vi "bapsf_motion_lv.vi"(4 "error in":errorcluster, 6 "Request data":variant, 7 "Request":string) -> (0 "error out":errorcluster, 2 "Response data":variant)   [LabVIEW 2018]
panel:
  out "Python session":refnum<k35>
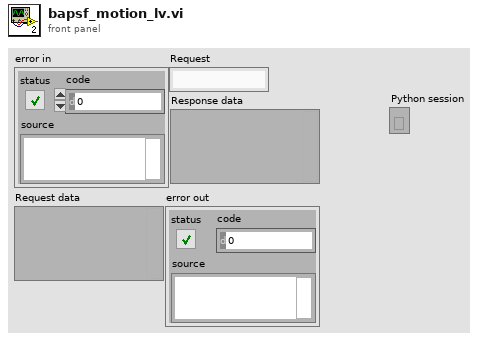
[diagram p1: front panel]
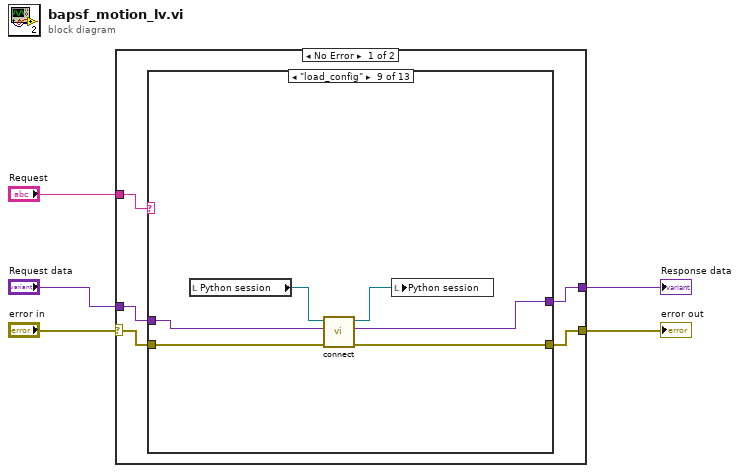
[diagram p0: block diagram]
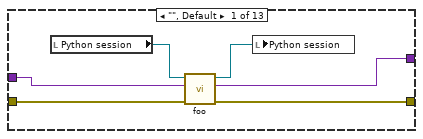
[diagram p2: hidden frame]
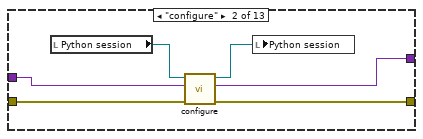
[diagram p3: hidden frame]
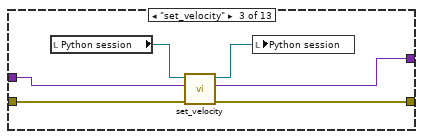
[diagram p4: hidden frame]
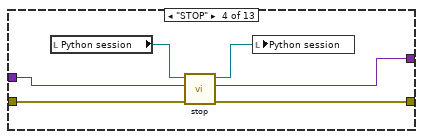
[diagram p5: hidden frame]
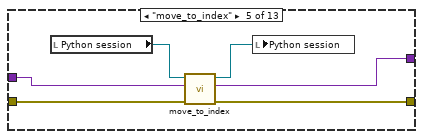
[diagram p6: hidden frame]
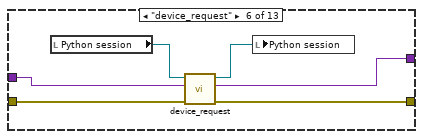
[diagram p7: hidden frame]
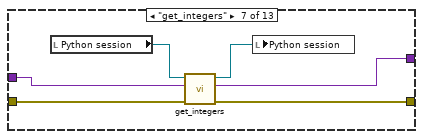
[diagram p8: hidden frame]
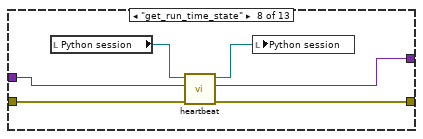
[diagram p9: hidden frame]
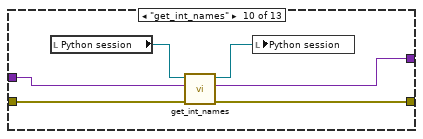
[diagram p10: hidden frame]
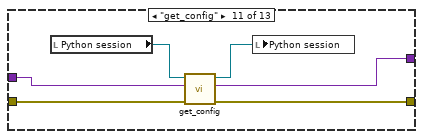
[diagram p11: hidden frame]
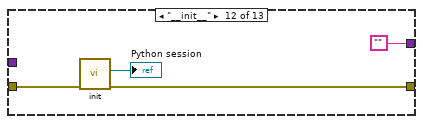
[diagram p12: hidden frame]
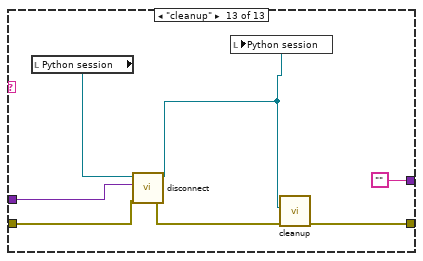
[diagram p13: hidden frame]
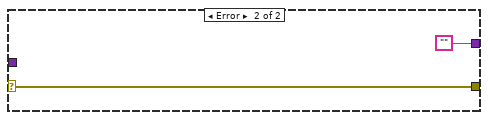
[diagram p14: hidden frame]
diagram:
  n1 = case shown="No Error" "error in" {
    selector: "error in" -> [w9 w89]
    tunnel: [w7 w89] -> w4
    tunnel: "Request" -> [w10 _]
    tunnel: "Request data" -> [w8 _]
    tunnel: [w6 ""] -> w1
    frame No Error {
      n2 = case shown="\"load_config\"" w10 {
        tunnel: w9 -> [w16 w22 w28 w34 w40 w46 w52 w58 w64 w70 w76 w79 w83]
        tunnel: w8 -> [w15 w21 w27 w33 w39 w45 w51 w57 w63 w69 w75 _ w84]
        tunnel: [w11 w18 w24 w30 w36 w42 w48 w54 w60 w66 w72 w78 w86] -> w7
        tunnel: [w12 w17 w23 w29 w35 w41 w47 w53 w59 w65 w71 "" ""] -> w6
        frame "", Default {
          n3 = local read "Python session"() -> (w14:refnum<k35>)
          n4 = call "foo.vi"("error in (no error)"=w16, "Request data"=w15, "Python session in"=w14) -> ("error out"=w11:errorcluster, "Response data"=w12:variant, "Python session out"=w13:refnum<k35>)  [unwired: 2 in]
          n5 = local write "Python session"(w13) -> ()
        }
        frame "configure" {
          n6 = local read "Python session"() -> (w20:refnum<k35>)
          n7 = call "configure.vi"("error in (no error)"=w22, "Request data"=w21, "Python session in"=w20) -> ("error out"=w18:errorcluster, "Response data"=w17:variant, "Python session out"=w19:refnum<k35>)  [unwired: 2 in]
          n8 = local write "Python session"(w19) -> ()
        }
        frame "set_velocity" {
          n9 = local read "Python session"() -> (w26:refnum<k35>)
          n10 = call "set_velocity.vi"("error in (no error)"=w28, "Request data"=w27, "Python session in"=w26) -> ("error out"=w24:errorcluster, "Response data"=w23:variant, "Python session out"=w25:refnum<k35>)  [unwired: 2 in]
          n11 = local write "Python session"(w25) -> ()
        }
        frame "STOP" {
          n12 = local read "Python session"() -> (w32:refnum<k35>)
          n13 = call "stop.vi"("error in (no error)"=w34, "Request data"=w33, "Python session in"=w32) -> ("error out"=w30:errorcluster, "Response data"=w29:variant, "Python session out"=w31:refnum<k35>)  [unwired: 2 in]
          n14 = local write "Python session"(w31) -> ()
        }
        frame "move_to_index" {
          n15 = local read "Python session"() -> (w38:refnum<k35>)
          n16 = call "move_to_index.vi"("error in (no error)"=w40, "Request data"=w39, "Python session in"=w38) -> ("error out"=w36:errorcluster, "Response data"=w35:variant, "Python session out"=w37:refnum<k35>)  [unwired: 2 in]
          n17 = local write "Python session"(w37) -> ()
        }
        frame "device_request" {
          n18 = local read "Python session"() -> (w44:refnum<k35>)
          n19 = call "device_request.vi"("error in (no error)"=w46, "Request data"=w45, "Python session in"=w44) -> ("error out"=w42:errorcluster, "Response data"=w41:variant, "Python session out"=w43:refnum<k35>)  [unwired: 2 in]
          n20 = local write "Python session"(w43) -> ()
        }
        frame "get_integers" {
          n21 = local read "Python session"() -> (w50:refnum<k35>)
          n22 = call "get_integers.vi"("error in (no error)"=w52, "Request data"=w51, "Python session in"=w50) -> ("error out"=w48:errorcluster, "Response data"=w47:variant, "Python session out"=w49:refnum<k35>)  [unwired: 2 in]
          n23 = local write "Python session"(w49) -> ()
        }
        frame "get_run_time_state" {
          n24 = local read "Python session"() -> (w56:refnum<k35>)
          n25 = call "heartbeat.vi"("error in (no error)"=w58, "Request data"=w57, "Python session in"=w56) -> ("error out"=w54:errorcluster, "Response data"=w53:variant, "Python session out"=w55:refnum<k35>)  [unwired: 2 in]
          n26 = local write "Python session"(w55) -> ()
        }
        frame "load_config" {
          n27 = local read "Python session"() -> (w62:refnum<k35>)
          n28 = call "connect.vi"("error in (no error)"=w64, "Request data"=w63, "Python session in"=w62) -> ("error out"=w60:errorcluster, "Response data"=w59:variant, "Python session out"=w61:refnum<k35>)  [unwired: 2 in]
          n29 = local write "Python session"(w61) -> ()
        }
        frame "get_int_names" {
          n30 = local read "Python session"() -> (w68:refnum<k35>)
          n31 = call "get_int_names.vi"("error in (no error)"=w70, "Request data"=w69, "Python session in"=w68) -> ("error out"=w66:errorcluster, "Response data"=w65:variant, "Python session out"=w67:refnum<k35>)  [unwired: 2 in]
          n32 = local write "Python session"(w67) -> ()
        }
        frame "get_config" {
          n33 = local read "Python session"() -> (w74:refnum<k35>)
          n34 = call "get_config.vi"("error in (no error)"=w76, "Request data"=w75, "Python session in"=w74) -> ("error out"=w72:errorcluster, "Response data"=w71:variant, "Python session out"=w73:refnum<k35>)  [unwired: 2 in]
          n35 = local write "Python session"(w73) -> ()
        }
        frame "__init__" {
          n36 = call "init.vi"("error in"=w79) -> ("error out"=w78:errorcluster, "Python session"=→"Python session":refnum<k35>)  [unwired: 5 in]
        }
        frame "cleanup" {
          n37 = local read "Python session"() -> (w85:refnum<k35>)
          n38 = call "disconnect.vi"("error in (no error)"=w83, "Request data"=w84, "Python session in"=w85) -> ("error out"=w82:errorcluster, "Python session out"=w81:refnum<k35>)  [unwired: 2 in, 1 out]
          n39 = local write "Python session"(w81) -> ()
          n40 = call "cleanup.vi"("error in"=w82, "Python session"=w81) -> ("error out"=w86:errorcluster)  [unwired: 5 in]
        }
      }
    }
    frame Error {
    }
  }
  "Response data" <- w1
  "error out" <- w4
